vi "QPlus_Data_Analyzer_beta.vi"(11 "File Path":path) -> (0 "Resonance Frequency":dbl, 1 "Quality Factor":dbl, 2 "FWHM":dbl, 3 "Integrated Signal":cluster{"Y":dbl[], "Y":dbl[]}[](graph))   [LabVIEW 2016]
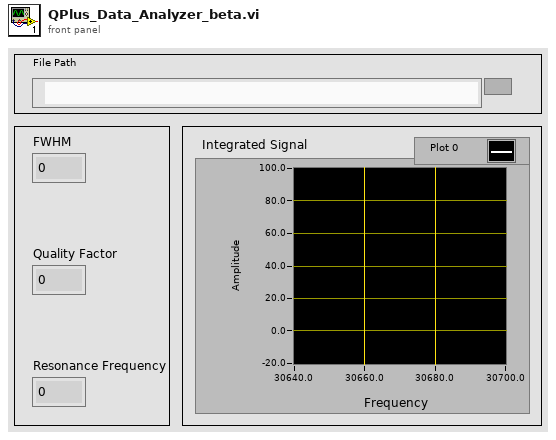
[diagram p1: front panel]
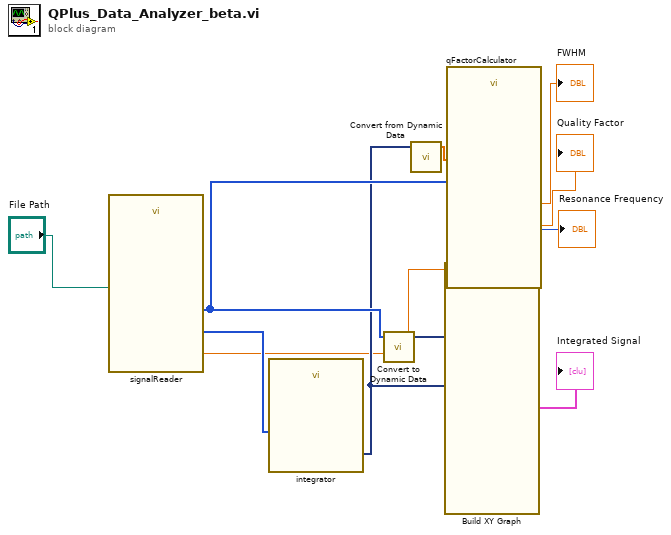
[diagram p0: block diagram]
diagram:
  n1 = call "signalReader.vi"("Filename"="File Path") -> ("Step Size"=w1:dbl, "Signal Column"=w11:i64[], "Frequency Column"=w8:i64[])  [unwired: 8 in]
  n2 = call "integrator.vi"("Signal"=w11) -> ("Result"=w6:dynamicdata)  [unwired: 10 in]
  n3 = call "Convert to Dynamic Data"("Array"=w8) -> ("Dynamic Data Type"=w9:dynamicdata)  [unwired: 3 in]
  n4 = call "Convert from Dynamic Data"("Dynamic Data Type"=w6) -> ("Array"=w5:dbl[])  [unwired: 3 in]
  n5 = call "Build XY Graph"("Y Input"=w6, "X Input"=w9) -> ("XY Graph"=→"Integrated Signal":cluster{"Y":dbl[], "Y":dbl[]}[])  [unwired: 3 in, 6 out]
  n6 = call "qFactorCalculator.vi"("Step Size"=w1, "Frequencies"=w8, "Signal"=w5) -> ("Resonance Frequency"=→"Resonance Frequency":i32, "FWHM"=→"FWHM":dbl, "Q-Factor"=→"Quality Factor":dbl)  [unwired: 6 in]
